vi "receive.vi"(8 "error in (no error)":errorcluster, 11 "Redis TCP Client in":refnum<class "Redis TCP Client.lvclass">) -> (0 "error out":errorcluster, 1 "timed out?":bool, 2 "RESP3 Value":variant, 3 "Redis TCP Client out":refnum<class "Redis TCP Client.lvclass">)   [LabVIEW 2019, in "Redis Client for LabVIEW.lvlib" / "Redis TCP Client.lvclass"]
uses:
  Redis TCP Client.lvclass
  Redis TCP Client.lvclass/Redis TCP Client.ctl
  lib/RESP3-for-LabVIEW/RESP3/RESP3 Parser/RESP3 Parser.lvclass
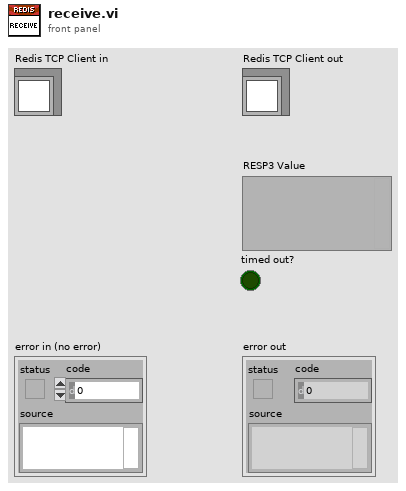
[diagram p1: front panel]
types:
  T1 = enum16{"Standard", "Buffered", "CRLF", "Immediate"}
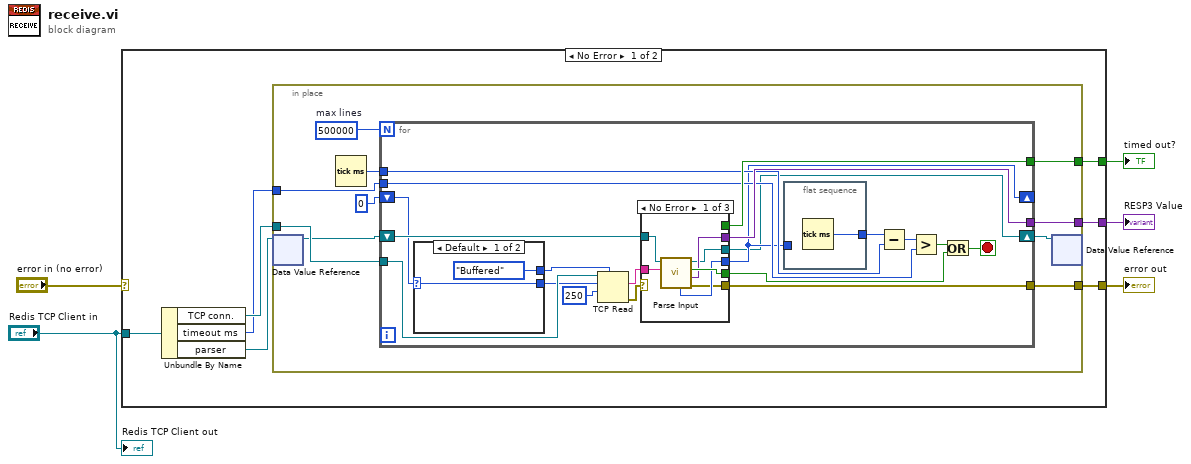
[diagram p0: block diagram]
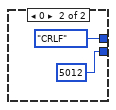
[diagram p2: hidden frame]
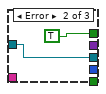
[diagram p3: hidden frame]
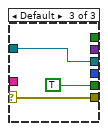
[diagram p4: hidden frame]
diagram:
  n1 = case shown="No Error" "error in (no error)" {
    selector: "error in (no error)" -> [_ w60]
    tunnel: "Redis TCP Client in" -> [w7 _]
    tunnel: [w10 _] -> w3
    tunnel: [w9 w60] -> w2
    tunnel: [w8 _] -> w1
    frame No Error {
      n2 = Unbundle By Name(w7) -> ("TCP conn."=w12:refnum<k5>, "timeout ms"=w11:i32, "parser"=w6:refnum<data-value>)
      n3 = in-place {
        in-place-border: w12 -> [w22]
        in-place-border: w11 -> [w21]
        in-place-border: [w20] -> w10
        in-place-border: [w19] -> w9
        in-place-border: [w18] -> w8
        w17 = 500000  # max lines
        n4 = in-place-dvr #1(w6) -> (w16:refnum<class "RESP3 Parser.lvclass">)  [unwired: 1 out]
        n5 = Tick Count (ms)() -> (millisecond timer value=w13:u32)
        n6 = for {
          N: w17 -> [_]
          tunnel: w22 -> [w42]
          tunnel: w21 -> [w28]
          tunnel: [w40] -> w20
          tunnel: [w39] -> w19
          tunnel: [w37] -> w18
          shift-right: [w23] -> w14
          shift-left: w16 -> [w36]
          shift-right: [w24] -> _
          shift-left: 0 ("bytes to read") -> [w35]
          tunnel: w13 -> [w30]
          stop <- w26 stop-if-true
          n7 = case shown="Default" w35 {
            selector: w35 -> [w44 _]
            tunnel: [T1."Buffered" ("mode (standard)") T1."CRLF" ("mode (standard)")] -> w34
            tunnel: [w44 5012 ("bytes to read")] -> w32
            frame Default {
            }
            frame 0 {
            }
          }
          n8 = TCP Read(connection ID=w42, bytes to read=w32, 7:w34, 9:250 ("timeout ms (25000)")) -> (data out=w38:string, error out=w41:errorcluster)  [unwired: 1 in, 1 out]
          n9 = case shown="No Error" w41 {
            selector: w41 -> [_ _ w59]
            tunnel: [_ TRUE _] -> w40
            tunnel: [w48 _ w59] -> w39
            tunnel: w38 -> [w53 _ _]
            tunnel: [w51 _ _] -> w37
            tunnel: w36 -> [w54 w55 w57]
            tunnel: [w52 _ TRUE ("finished?")] -> w33
            tunnel: [w50 _ _] -> w24
            tunnel: [w49 w55 w57] -> w23
            frame No Error {
              n10 = call-dynamic "Parse Input.vi"("input line"=w53, "RESP3 Parser in"=w54) -> ("error out"=w48:errorcluster, "RESP3 Value"=w51:variant, "finished?"=w52:bool, "RESP3 Parser out"=w49:refnum<class "RESP3 Parser.lvclass">, "next bytes"=w50:i32)  [unwired: 5 in]
            }
            frame Error {
            }
            frame Default {
            }
          }
          n11 = flat-sequence {
            tunnel: [w43] -> w31
            tunnel: w24 -> [_]
            frame #0 {
              n12 = Tick Count (ms)() -> (millisecond timer value=w43:u32)
            }
          }
          n13 = Subtract(x=w31, y=w30) -> (x-y=w29:u32)
          n14 = Greater?(x=w29, y=w28) -> (0:w25:bool)
          n15 = Or(x=w25, y=w33) -> (x .or. y?=w26:bool)
        }
        n16 = in-place-dvr #1(w14) -> ()  [unwired: 2 out]
      }
    }
    frame Error {
    }
  }
  "error out" <- w2
  "RESP3 Value" <- w1
  "timed out?" <- w3
  "Redis TCP Client out" <- "Redis TCP Client in"
